vi "创建URL字符串.vi"(2 "参数":string[](array[string]), 3 "初始URL":string) -> (1 "结果URL":string)   [LabVIEW 2014]
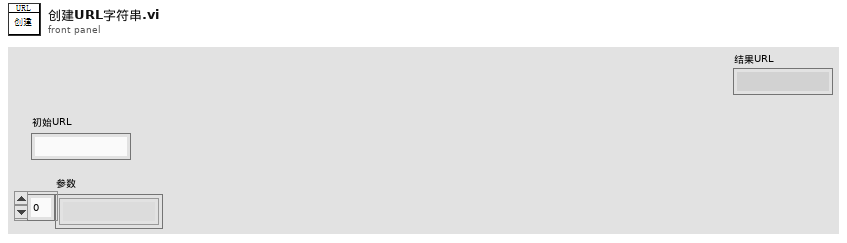
[diagram p1: front panel]
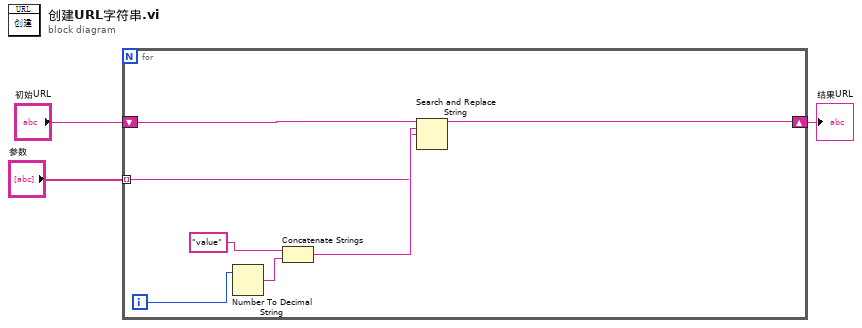
[diagram p0: block diagram]
diagram:
  n1 = for {
    tunnel: "参数" -> [w5] mode=indexing
    shift-right: [w4] -> w1
    shift-left: "初始URL" -> [w10]
    i -> [w8]
    n2 = Number To Decimal String(number=w8) -> (decimal integer string=w7:string)  [unwired: 1 in]
    n3 = Concatenate Strings("value", w7) -> (w6:string)
    n4 = Search and Replace String(input string=w10, search string=w6, replace string=w5) -> (result string=w4:string)  [unwired: 5 in, 3 out]
  }
  "结果URL" <- w1
